vi "PCert-ConfigPageNF-AccessorActAddr.vi"(8 "error in (no error)":errorcluster, 11 "ERP-ConfigPageNF in":refnum<class "PCert-ConfigPageNF.lvclass">) -> (0 "error out":errorcluster, 2 "Actor Address":string, 3 "ERP-ConfigPageNF out":refnum<class "PCert-ConfigPageNF.lvclass">)   [LabVIEW 2013, in "PCert-ConfigPageNF.lvclass"]
uses:
  PCert-ConfigPageNF.lvclass
  PCert-ConfigPageNF.lvclass/PCert-ConfigPageNF.ctl
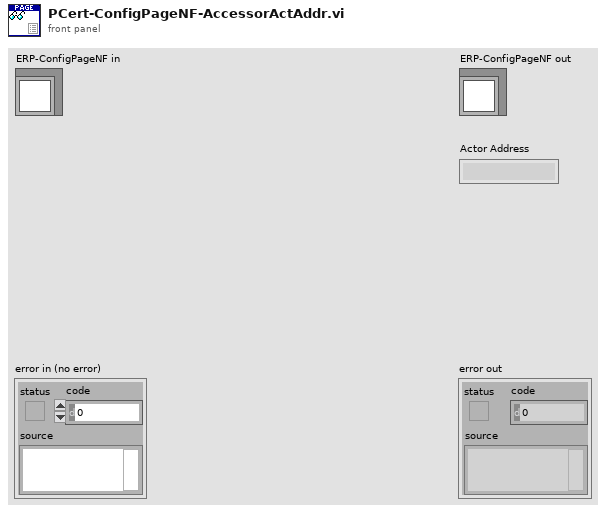
[diagram p1: front panel]
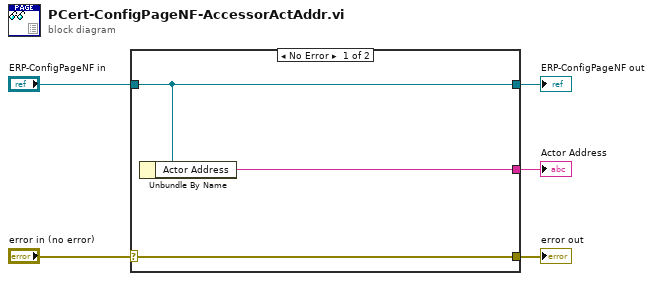
[diagram p0: block diagram]
diagram:
  n1 = case shown="No Error" "error in (no error)" {
    selector: "error in (no error)" -> [w8 w9]
    tunnel: [w8 w9] -> w4
    tunnel: [w7 w10] -> w2
    tunnel: "ERP-ConfigPageNF in" -> [w7 w10]
    tunnel: [w6 _] -> w1
    frame No Error {
      n2 = Unbundle By Name(w7) -> ("Actor Address"=w6:string)
    }
    frame Error {
    }
  }
  "error out" <- w4
  "ERP-ConfigPageNF out" <- w2
  "Actor Address" <- w1
